vi "Configure Output Impedance.vi"(8 "error in (no error)":errorcluster, 10 "Impedance (1: High Impedance)":i32(ring)=1 items=["50 Ohms", "High Impedance"], 11 "VISA resource name":refnum<visa-resource-name>) -> (0 "error out":errorcluster, 3 "VISA resource name out":refnum<visa-resource-name>)   [LabVIEW 2017, in "Scope.lvlib" / "Tektronix DPO MSO 2000 4000 Series.lvlib"]
doc: "Configures the Arbitrary Function Generator output load impedance.\n\n<B>Notes:</B>\n(1) This VI is available for MDO3000 Series only.\n\n(2) Requires the MDO3AFG option to be installed."
uses:
  Tektronix DPO MSO 2000 4000 Series.lvlib
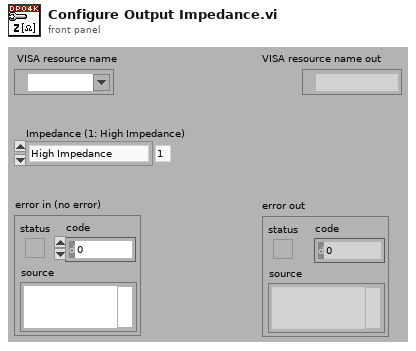
[diagram p1: front panel]
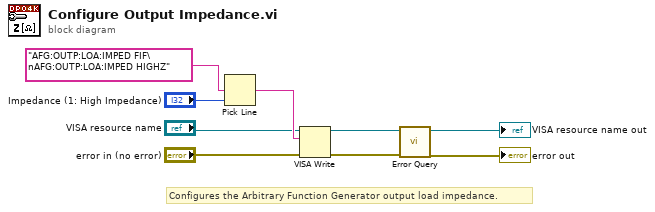
[diagram p0: block diagram]
diagram:
  # "Configures the Arbitrary Function Generator output load impedance."
  n1 = Pick Line(multi-line string="AFG:OUTP:LOA:IMPED FIF\nAFG:OUTP:LOA:IMPED HIGHZ", line index="Impedance (1: High Impedance)") -> (output string=w7:string)  [unwired: 1 in]
  n2 = VISA Write(VISA resource name="VISA resource name", write buffer=w7, error in (no error)="error in (no error)") -> (VISA resource name out=w5:refnum<visa-resource-name>, error out=w4:errorcluster)  [unwired: 1 out]
  n3 = call "Error Query.vi"("error in (no error)"=w4, "VISA resource name"=w5) -> ("error out"=→"error out":errorcluster, "VISA resource name out"=→"VISA resource name out":refnum<visa-resource-name>)  [unwired: 6 in, 2 out]
